vi "SVFA Frequency Response (Mag-Phase).vi"   [LabVIEW 2017]
doc: "Computes the magnitude, phase, and coherence of the frequency response of the device under test [DUT]. This VI computes the ratio of the output to the input of the DUT. Wire data to the <B>stimulus signal X [Eux]</B> and <B>response signal Y [Euy]</B> inputs to determine the polymorphic instance to use or manually select the instance."
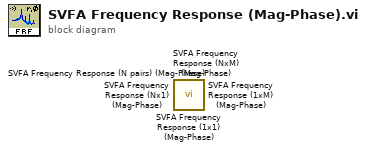
[diagram p0: block diagram]
diagram:
  n1 = call <vilib>:"SVFA Frequency Response (1x1) (Mag-Phase).vi"() -> ()  [unwired: 11 in, 9 out]
  n2 = call <vilib>:"SVFA Frequency Response (NxM) (Mag-Phase).vi"() -> ()  [unwired: 11 in, 9 out]
  n3 = call <vilib>:"SVFA Frequency Response (Nx1) (Mag-Phase).vi"() -> ()  [unwired: 11 in, 9 out]
  n4 = call <vilib>:"SVFA Frequency Response (1xM) (Mag-Phase).vi"() -> ()  [unwired: 11 in, 9 out]
  n5 = call <vilib>:"SVFA Frequency Response (N pairs) (Mag-Phase).vi"() -> ()  [unwired: 11 in, 9 out]
